vi "midiOutPatchChange.vi"(8 "error in":errorcluster, 10 "Patch":u32, 11 "midi in":refnum<class "midi.lvclass">) -> (0 "error out":errorcluster, 3 "midi out":refnum<class "midi.lvclass">)   [LabVIEW 2020, in "midi.lvclass"]
uses:
  midi.lvclass
  midi.lvclass/midi.ctl
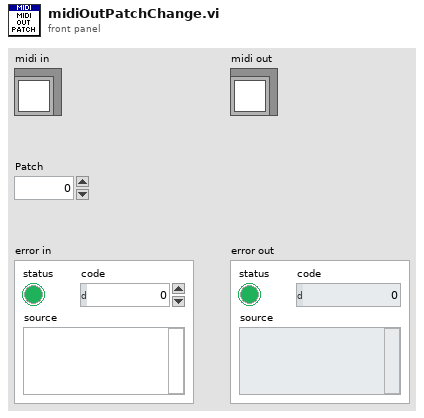
[diagram p1: front panel]
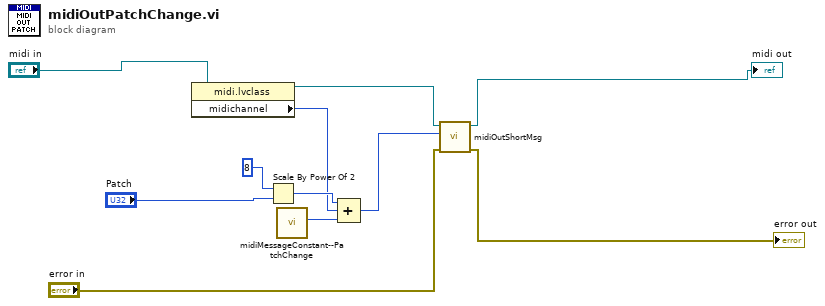
[diagram p0: block diagram]
diagram:
  n1 = property class="midi.lvclass"(reference="midi in") -> (reference out=w4:refnum<class "midi.lvclass">, "midichannel"=w2:u64)  [unwired: 1 in, 1 out]
  n2 = Scale By Power Of 2(n=8, x="Patch") -> (x*2^n=w8:u32)
  n3 = call "midiMessageConstant--PatchChange.vi"() -> ("Message"=w3:u8)  [unwired: 11 in]
  n4 = Compound Arithmetic op=ADD(w8, w2, w3) -> (w6:u64)
  n5 = call "midiOutShortMsg.vi"("error in"="error in", "data"=w6, "midi in"=w4) -> ("error out"=→"error out":errorcluster, "midi out"=→"midi out":refnum<class "midi.lvclass">)  [unwired: 7 in]
